vi "Configure.vi"(8 "error in (no error)":errorcluster caption="错误输入（无错误）", 10 "Function":T1, 11 "TH6402 输入":refnum<class "TH6402.lvclass">) -> (0 "error out":errorcluster caption="错误输出", 3 "TH6402 输出":refnum<class "TH6402.lvclass">)   [LabVIEW 2020, in "DP.lvlib" / "TH6402.lvclass"]
uses:
  TH6402.lvclass
  D:/LVProject/Class/LVDevClass/DP/root/DP.lvclass
  root/Function.ctl
  TH6402.lvclass/TH6402.ctl
  root/DP.lvclass
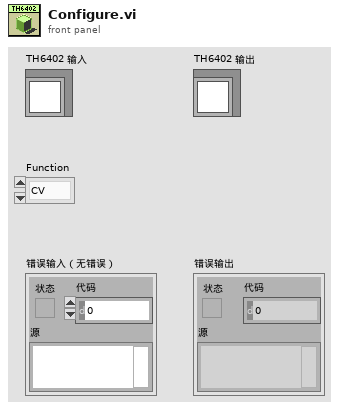
[diagram p1: front panel]
types:
  T1 = typedef "DP.lvlib/DP.lvclass/Function.ctl" = enum16{"CV", "CC"}
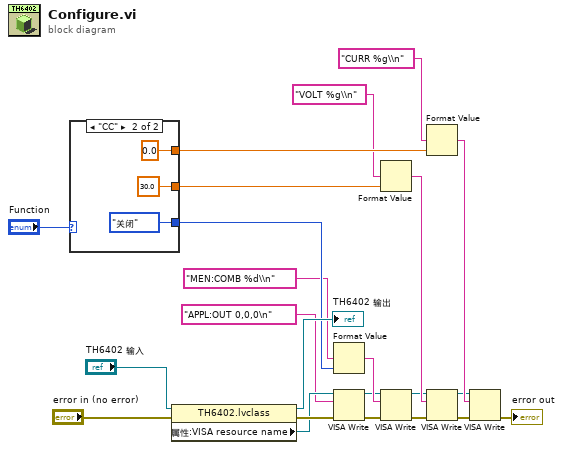
[diagram p0: block diagram]
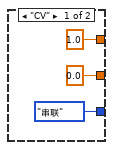
[diagram p2: hidden frame]
diagram:
  n1 = case shown="\"CC\"" "Function" {
    tunnel: [enum16{"关闭", "串联", "并联"}."串联" ("通道组合") enum16{"关闭", "串联", "并联"}."关闭" ("通道组合")] -> w18
    tunnel: [0.0 30.0] -> w17
    tunnel: [1.0 0.0] -> w12
    frame "CV" {
    }
    frame "CC" {
    }
  }
  n2 = property class="TH6402.lvclass"(reference="TH6402 输入", error in="error in (no error)") -> (reference out=→"TH6402 输出":refnum<class "TH6402.lvclass">, error out=w8:errorcluster, "属性:VISA resource name"=w3:refnum<visa-resource-name>)
  n3 = Format Value(format string="MEN:COMB %d\\n" ("格式字符串"), value (0)=w18) -> (output string=w20:string)  [unwired: 1 in]
  n4 = VISA Write(VISA resource name=w3, write buffer="APPL:OUT 0,0,0\n" ("写入缓冲区"), error in (no error)=w8) -> (VISA resource name out=w2:refnum<visa-resource-name>, error out=w4:errorcluster)  [unwired: 1 out]
  n5 = Format Value(format string="VOLT %g\\n" ("格式字符串"), value (0)=w17) -> (output string=w16:string)  [unwired: 1 in]
  n6 = VISA Write(VISA resource name=w2, write buffer=w20, error in (no error)=w4) -> (VISA resource name out=w15:refnum<visa-resource-name>, error out=w9:errorcluster)  [unwired: 1 out]
  n7 = Format Value(format string="CURR %g\\n" ("格式字符串"), value (0)=w12) -> (output string=w14:string)  [unwired: 1 in]
  n8 = VISA Write(VISA resource name=w15, write buffer=w16, error in (no error)=w9) -> (VISA resource name out=w13:refnum<visa-resource-name>, error out=w10:errorcluster)  [unwired: 1 out]
  n9 = VISA Write(VISA resource name=w13, write buffer=w14, error in (no error)=w10) -> (error out=→"error out":errorcluster)  [unwired: 2 out]
